vi "ICNC Parameters Dlg.vi"(7 "AutoSaveFileName":string, 8 "error in (no error)":errorcluster caption="entrée d'erreur (pas d'erreur)", 9 "DisplayBasicButton":i32, 10 "DisplayLoadButton":i32, 11 "DisplaSaveButton":i32) -> (0 "error out":errorcluster caption="sortie d'erreur", 3 "function return":u32, 5 "AutoSaveFileName out":string)   [LabVIEW 2017, in "ICNC2.lvlib"]
doc: "DWORD ICNC_ParametersDlg ( int DisplaSaveButton,\n int DisplayLoadButton,\n int DisplayBasicButton,\n PCHAR AutoSaveFileName);"
uses:
  ICNC2.lvlib
  <userlib>/ICNC/ICNC2.dll
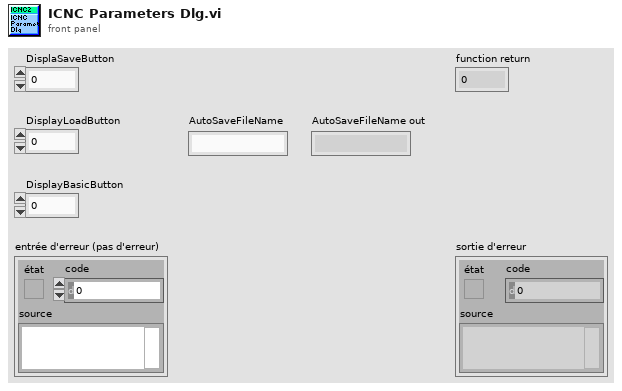
[diagram p1: front panel]
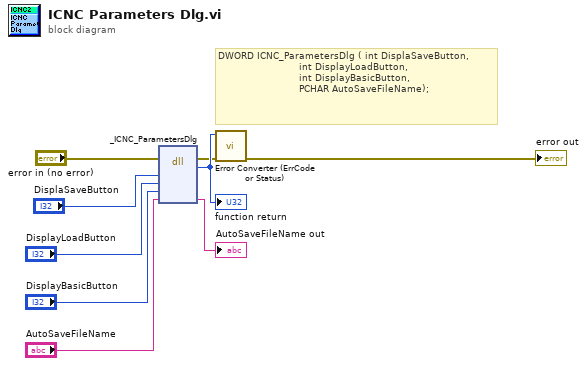
[diagram p0: block diagram]
diagram:
  # "DWORD ICNC_ParametersDlg ( int DisplaSaveButton,\n                           int DisplayLoadButton,\n                           int DisplayBasicButton,\n                           PCHAR AutoSaveFileName);"
  n1 = dll-call lib="C:/Program Files (x86)/National Instruments/LabVIEW 2017/user.lib/ICNC/ICNC2.*" fn="_ICNC_ParametersDlg"(error in="error in (no error)", "DisplaSaveButton"="DisplaSaveButton", "DisplayLoadButton"="DisplayLoadButton", "DisplayBasicButton"="DisplayBasicButton", "AutoSaveFileName"="AutoSaveFileName") -> (error out=w2:errorcluster, w9:u32, "AutoSaveFileName"=→"AutoSaveFileName out":string)  [unwired: 5 in, 1 out]
  "function return" <- w9
  n2 = call "Error Converter (ErrCode or Status).vi"("error in (no error)"=w2, "error code"=w9) -> ("error out"=→"error out":errorcluster)  [unwired: 9 in]
